vi "Batch_ListBuildSpecProjects.vi"(8 "error in (no error)":errorcluster, 11 "CommandLine":string[](array[string])) -> (0 "error out":errorcluster, 2 "test details":string, 3 "output to action":string)   [LabVIEW 2017]
uses:
  _lvcicd/_lvcicd_support_2017.lvlib
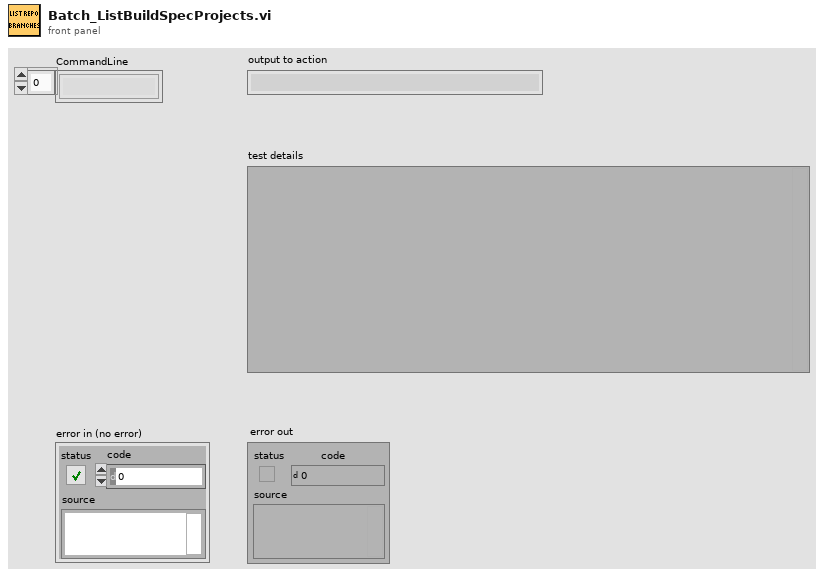
[diagram p1: front panel]
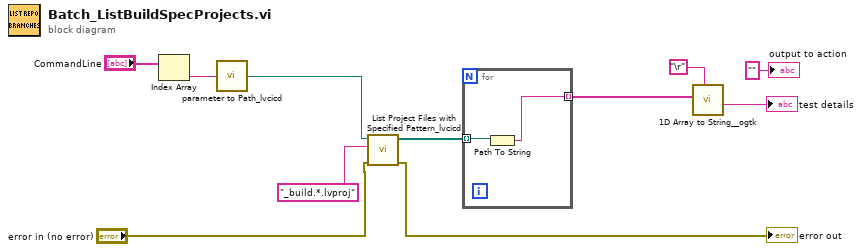
[diagram p0: block diagram]
diagram:
  n1 = Index Array(array="CommandLine") -> (element=w8:string)  [unwired: 1 in]
  n2 = call "parameter to Path_lvcicd.vi"("String"=w8) -> ("Path"=w11:path)
  n3 = call "List Project Files with Specified Pattern_lvcicd.vi"("error in (no error)"="error in (no error)", "pattern"="_build.*.lvproj", "Path"=w11) -> ("error out"=→"error out":errorcluster, "All Files in Dir"=w4:path[])  [unwired: 6 in, 1 out]
  n4 = for {
    tunnel: w4 -> [w13] mode=indexing
    tunnel: [w12] -> w3 mode=indexing
    n5 = Path To String(path=w13) -> (string=w12:string)
  }
  n6 = call <userlib>:"1D Array to String__ogtk.vi"("delimiter (Tab)"="\r", "Array of Strings"=w3) -> ("delimited string"=→"test details":string)  [unwired: 9 in]
  "output to action" <- "" ("output to action")
